vi "fire_logger_event.vi"(4 "user event":refnum<user-event>, 5 "Event Data":cluster{"level":i32, "message":string}, 6 "Control Ref":refnum<k24>, 7 "Event Common Data":T1) -> ()   [LabVIEW 2014]
uses:
  SwabianInstruments.TimeTagger
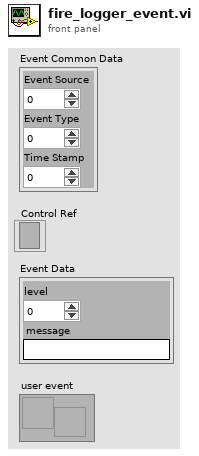
[diagram p1: front panel]
types:
  T1 = cluster{"Event Source":i32, "Event Type":u32, "Time Stamp":u32}
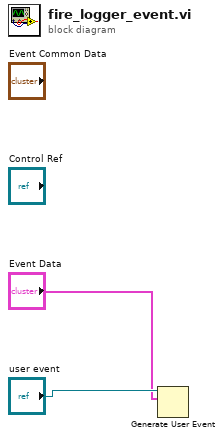
[diagram p0: block diagram]
diagram:
  n1 = Generate User Event(user event="user event", event data cluster="Event Data") -> ()  [unwired: 2 in, 2 out]
